vi "Robot Parameters.vi"() -> ()   [LabVIEW 2018]
panel:
  in  "LIDAR position y":dbl=0.06
  in  "LIDAR position x":dbl
  in  "gear ratio":dbl=86.3
  in  "center of mass y":dbl
  in  "center of mass x":dbl
  in  "robot length":dbl=0.25
  in  "robot width":dbl=0.25
  in  "wheel width":dbl=0.04
  in  "wheel radius":dbl=0.0768
  in  "inertia (Izz)":dbl=1.16
  in  "mass":dbl=43.5
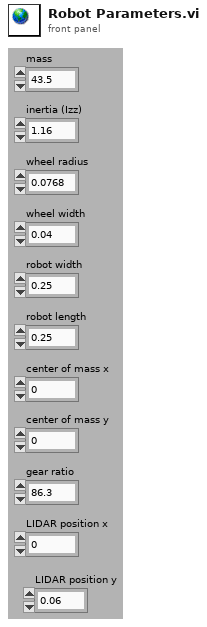
[diagram p1: front panel]
diagram:
